vi "21_DC Motor_PID_test.vi"() -> ()   [LabVIEW 2018]
uses:
  <userlib>/KNR OS 4.0 LabVIEW Toolkit/Type Definition/Resource.ctl
  <userlib>/KNR OS 4.0 LabVIEW Toolkit/Type Definition/DC Motor Port.ctl
panel:
  out "Desire Velosity (cm/sec)":dbl
  in  "switch":bool
  in  "Port":T1=4 items=["DS1"=4, "DS2"=5, "DS3"=6, "DS4"=7]
  out "Velocity (cm/sec) Chart":dbl(graph)
  out "Speed (+-100%)":dbl
  in  "Kd":dbl(slide)=0.01 scale=0.0..0.02
  in  "Ki":dbl(slide)=0.048 scale=0.0..0.2
  in  "Kp":dbl(slide)=0.2 scale=0.0..1.0
  in  "IP":string(combo)="172.22.11.2"
  in  "Resource":T2=enum."KNRm_DDDD"
  in  "stop":bool
  in  "Enable Motor":bool
  out "Position cm":dbl
  out "Velocity (cm/sec)":dbl
  in  "Reverse?":bool
  in  "Reset":bool
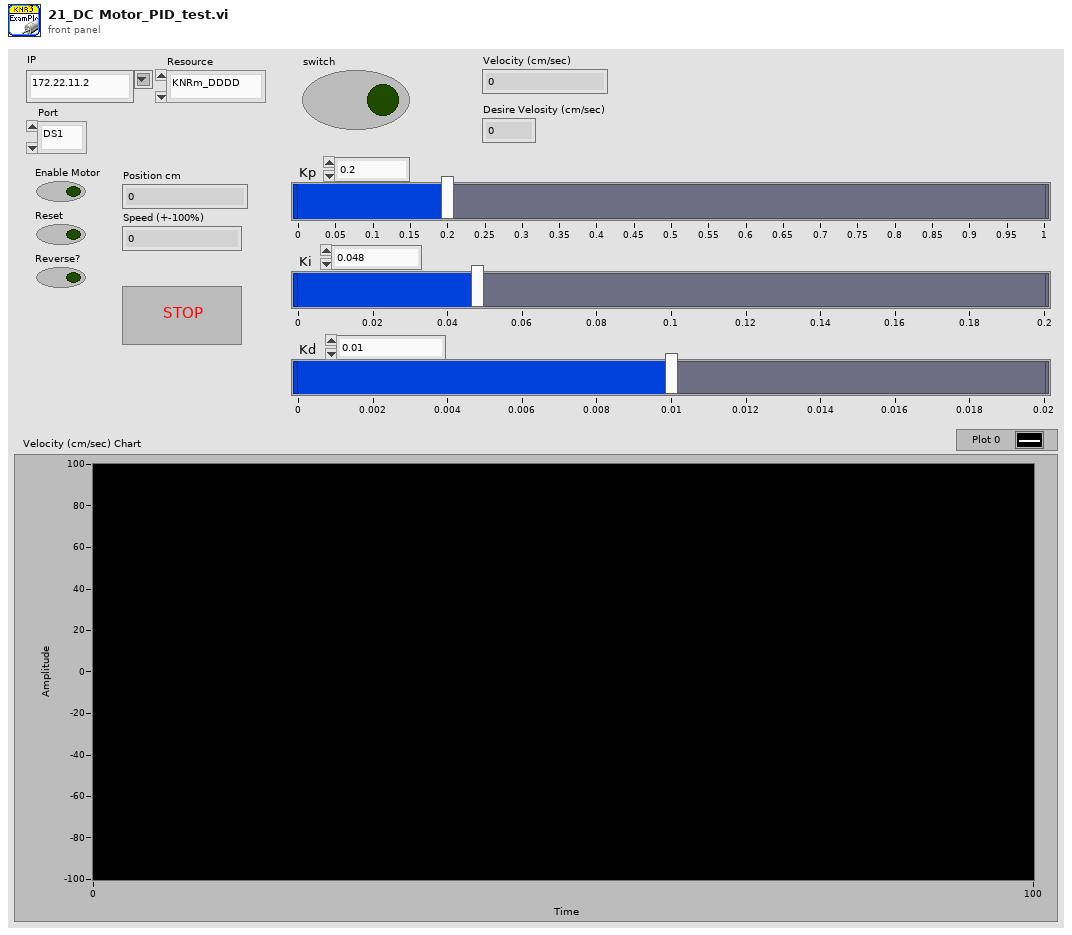
[diagram p1: front panel]
types:
  T1 = typedef "DC Motor Port.ctl" = u16
  T2 = typedef "Resource.ctl" = enum16{"KNRm_DDRC", "KNRm_DDDD", "KNRm_DDDR", "KNRm_DDDC", "KNR", "KNRm_neww"}
  T3 = typedef "KNR3 Reference.ctl" = cluster{"FPGA Session":refnum<class "FPGA Interface Base.lvclass">, "Resource":T2}
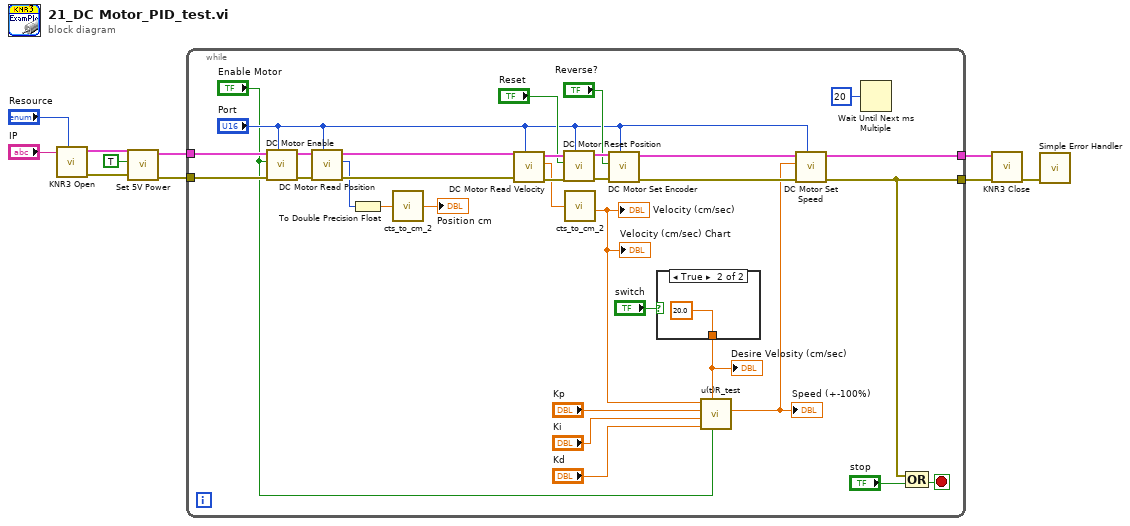
[diagram p0: block diagram]
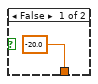
[diagram p2: hidden frame]
diagram:
  n1 = call <userlib>:"KNR3 Open.vi"("Resource"="Resource", "IP"="IP") -> ("error out"=w4:errorcluster, "KNR out"=w6:T3)  [unwired: 8 in]
  n2 = call <userlib>:"Set 5V Power.vi"("error in (no error)"=w4, "5V Power(T)"=TRUE ("5V Power"), "KNR in"=w6) -> ("error out"=w8:errorcluster, "KNR out"=w9:T3)  [unwired: 7 in]
  n3 = while {
    tunnel: w9 -> [w42]
    tunnel: w8 -> [w41]
    tunnel: [w20] -> w2
    tunnel: [w19] -> w1
    stop <- w39 stop-if-true
    n4 = call <userlib>:"DC Motor Enable.vi"("Port (DS1)"="Port", "error in (no error)"=w41, "Enable Motor(F)"="Enable Motor", "KNR in"=w42) -> ("error out"=w24:errorcluster, "KNR out"=w25:T3)  [unwired: 6 in]
    n5 = call <userlib>:"DC Motor Read Position.vi"("Port (DS1)"="Port", "error in (no error)"=w24, "KNR in"=w25) -> ("error out"=w36:errorcluster, "Position"=w27:i32, "KNR out"=w37:T3)  [unwired: 6 in]
    n6 = To Double Precision Float(number=w27) -> (double precision float=w26:dbl)
    n7 = call "cts_to_cm_2.vi"("cts"=w26) -> ("cm"=→"Position cm":dbl)
    n8 = call <userlib>:"DC Motor Read Velocity.vi"("Port (DS1)"="Port", "error in (no error)"=w36, "KNR in"=w37) -> ("error out"=w32:errorcluster, "Velocity (cts/sec)"=w31:dbl, "KNR out"=w35:T3)  [unwired: 6 in]
    n9 = call <userlib>:"DC Motor Reset Position.vi"("Port (DS1)"="Port", "error in (no error)"=w32, "Reset(F)"="Reset", "KNR in"=w35) -> ("error out"=w33:errorcluster, "KNR out"=w34:T3)  [unwired: 6 in]
    n10 = call "cts_to_cm_2.vi"("cts"=w31) -> ("cm"=w13:dbl)
    "Velocity (cm/sec)" <- w13
    "Velocity (cm/sec) Chart" <- w13
    n11 = call <userlib>:"DC Motor Set Encoder.vi"("Port (DS1)"="Port", "error in (no error)"=w33, "Reverse?(F)"="Reverse?", "KNR in"=w34) -> ("error out"=w22:errorcluster, "KNR out"=w23:T3)  [unwired: 6 in]
    n12 = case shown="True" "switch" {
      tunnel: [-20.0 20.0] -> w11
      frame False {
      }
      frame True {
      }
    }
    "Desire Velosity (cm/sec)" <- w11
    n13 = call "u(t)R_test.vi"("enable"="Enable Motor", "Desire Velosity"=w11, "Kd"="Kd", "Ki"="Ki", "Kp"="Kp", "Velocity"=w13) -> ("u(t)"=w14:dbl)  [unwired: 5 in]
    "Speed (+-100%)" <- w14
    n14 = call <userlib>:"DC Motor Set Speed.vi"("Port (DS1)"="Port", "error in (no error)"=w22, "Speed (+-100%)"=w14, "KNR in"=w23) -> ("error out"=w19:errorcluster, "KNR out"=w20:T3)  [unwired: 6 in]
    n15 = Wait Until Next ms Multiple(millisecond multiple=u32 20) -> ()  [unwired: 1 out]
    n16 = Compound Arithmetic op=OR(w19, "stop") -> (w39:bool)
  }
  n17 = call <userlib>:"KNR3 Close.vi"("error in (no error)"=w1, "KNR in"=w2) -> ("error out"=w7:errorcluster)  [unwired: 9 in]
  n18 = call <vilib>:"Simple Error Handler.vi"("error in (no error)"=w7) -> ()  [unwired: 4 in, 5 out]
